vi "Func_DropMultiTypeVIs.vi"(8 "error in":errorcluster, 11 "Control Path":path=path "C:/Users/dsmith.AMER/Desktop/ctl1.ctl") -> (0 "error out":errorcluster)   [LabVIEW 2010, in "TemplateGenerator.lvlib"]
uses:
  TemplateGenerator.lvlib
  <vilib>/Utility/traverseref.llb/VI Scripting - Traverse.lvlib
  <vilib>/Utility/traverseref.llb/TRef TravTarget.ctl
  <vilib>/Utility/miscctls.llb/LVPointTypeDef.ctl
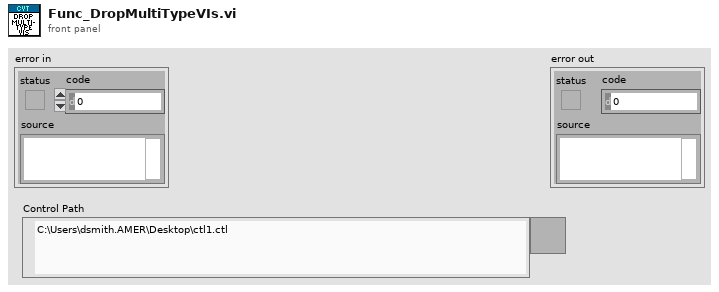
[diagram p1: front panel]
types:
  T1 = typedef "TRef TravTarget.ctl" = enum16{"FP", "BD", "Other"}
  T2 = typedef "LVPointTypeDef.ctl" = cluster{"Horizontal":i16, "Vertical":i16}
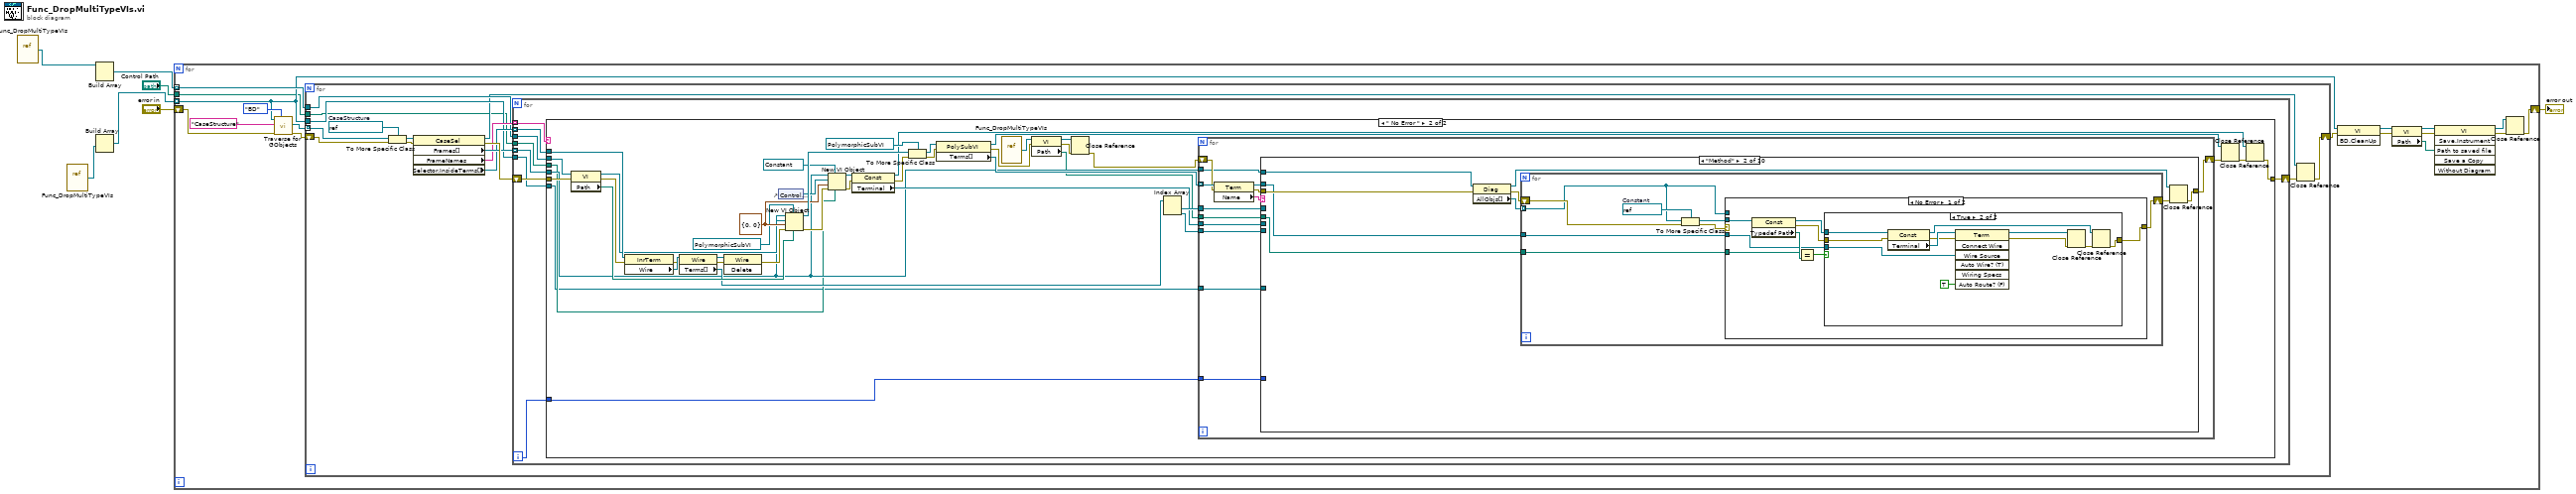
[diagram p0: block diagram]
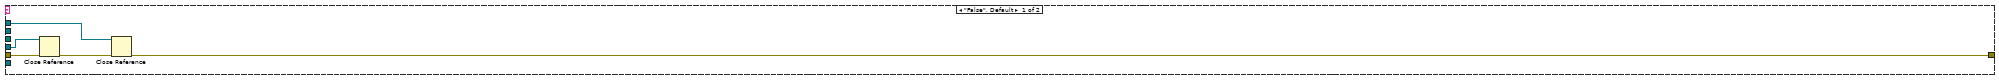
[diagram p2: hidden frame]
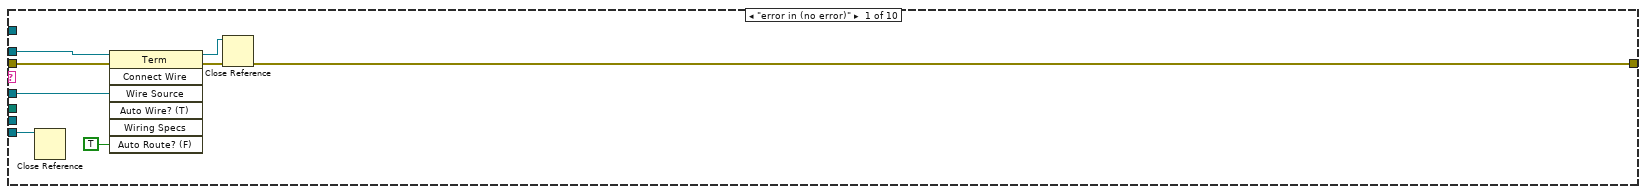
[diagram p3: hidden frame]
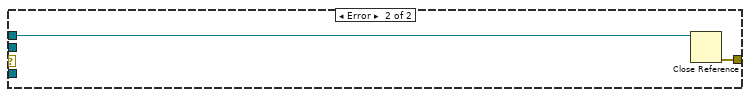
[diagram p5: hidden frame]
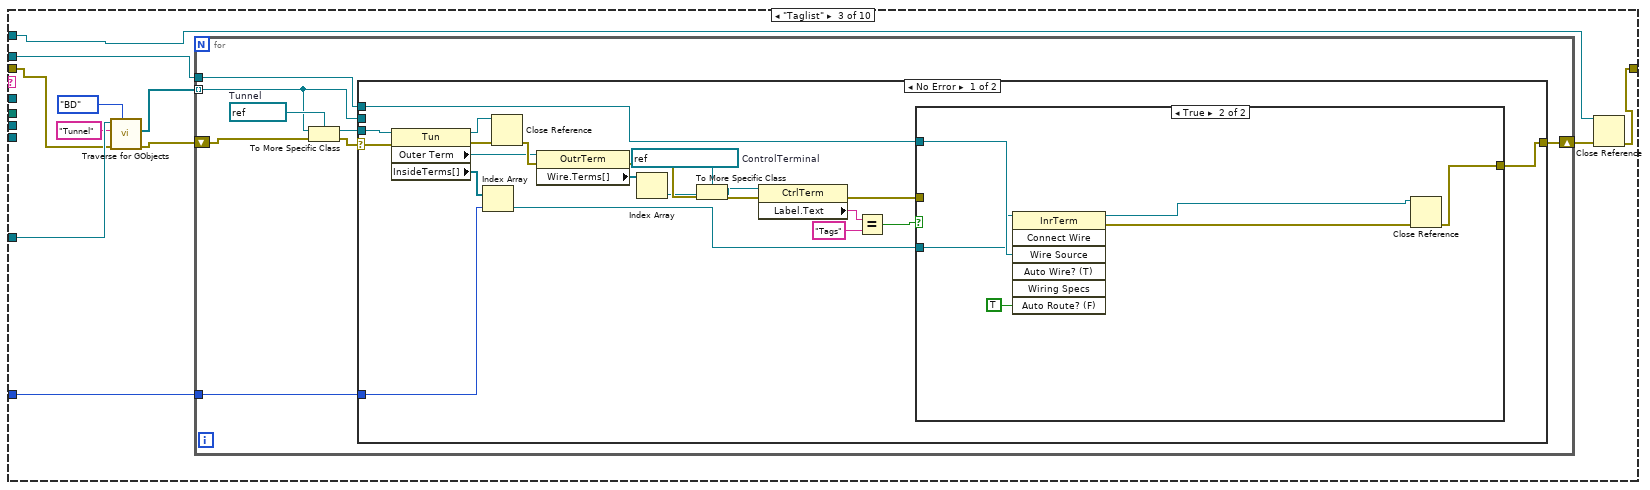
[diagram p6: hidden frame]
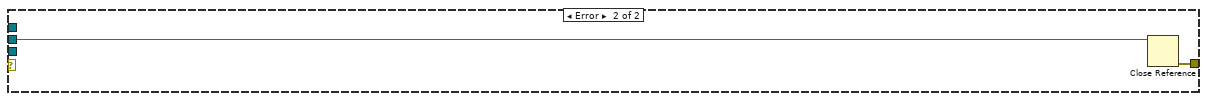
[diagram p8: hidden frame]
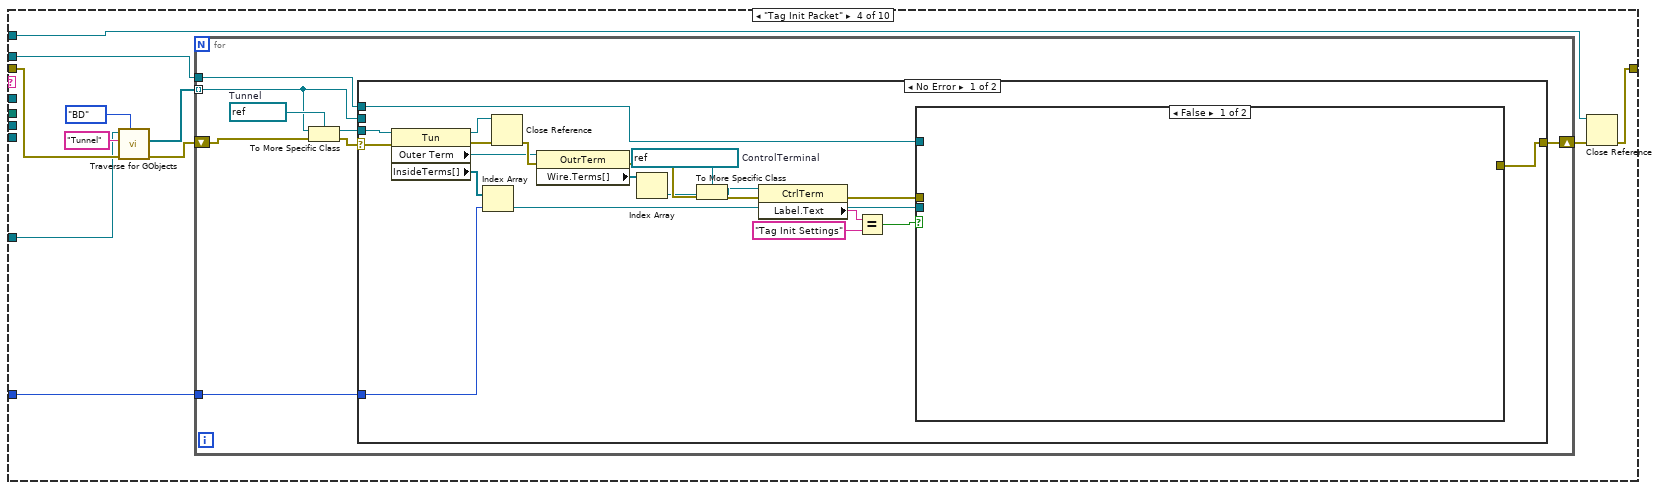
[diagram p9: hidden frame]
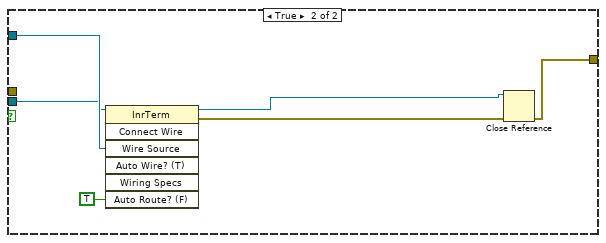
[diagram p10: hidden frame]
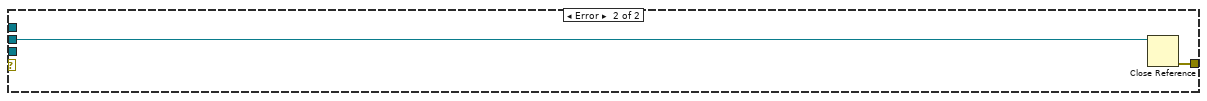
[diagram p11: hidden frame]
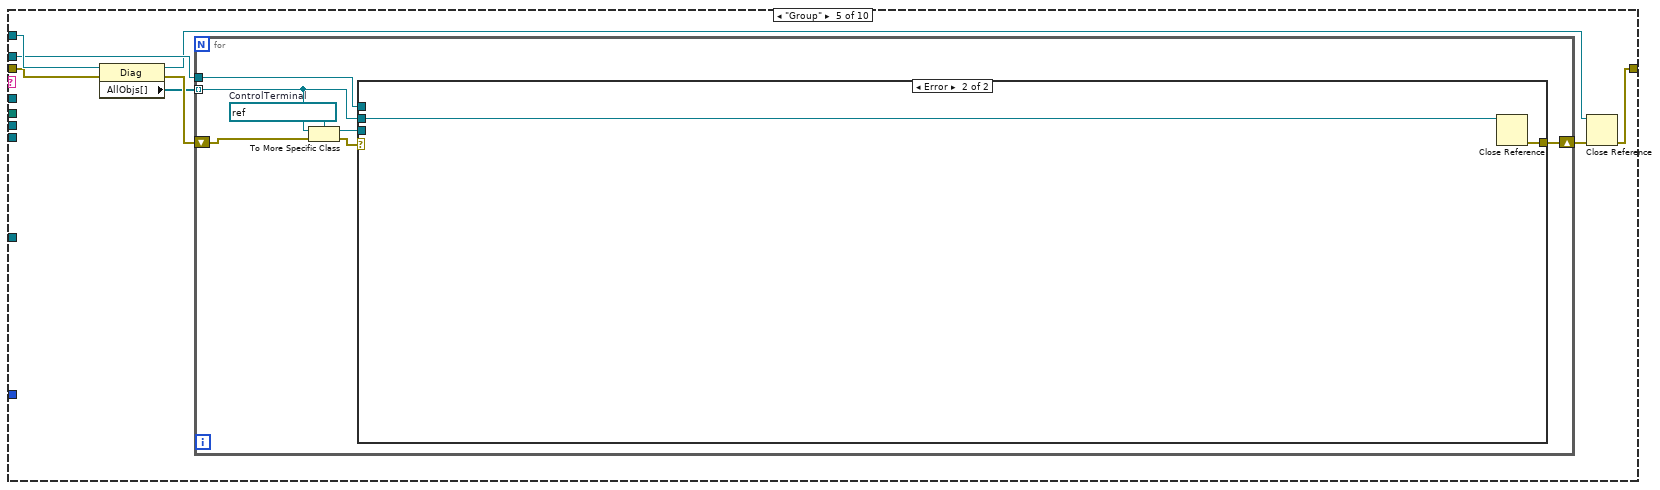
[diagram p12: hidden frame]
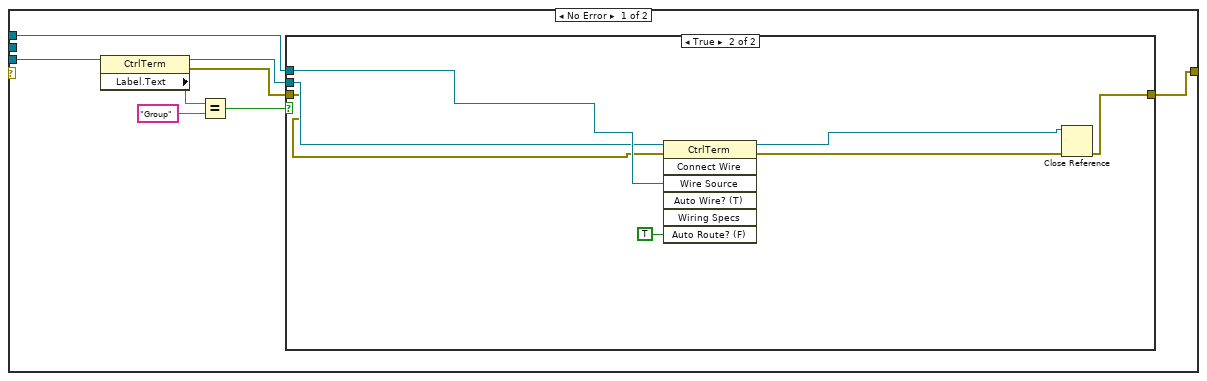
[diagram p13: hidden frame]
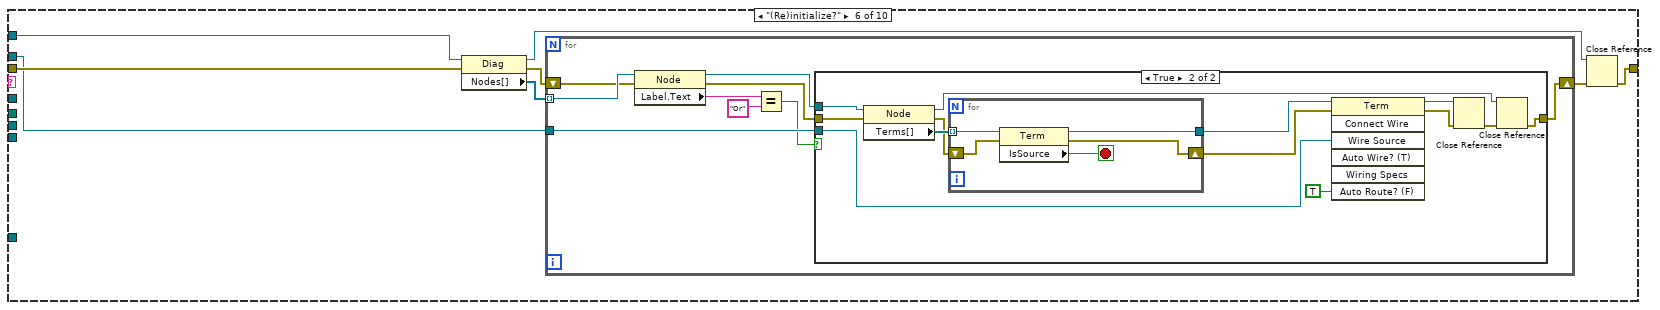
[diagram p15: hidden frame]
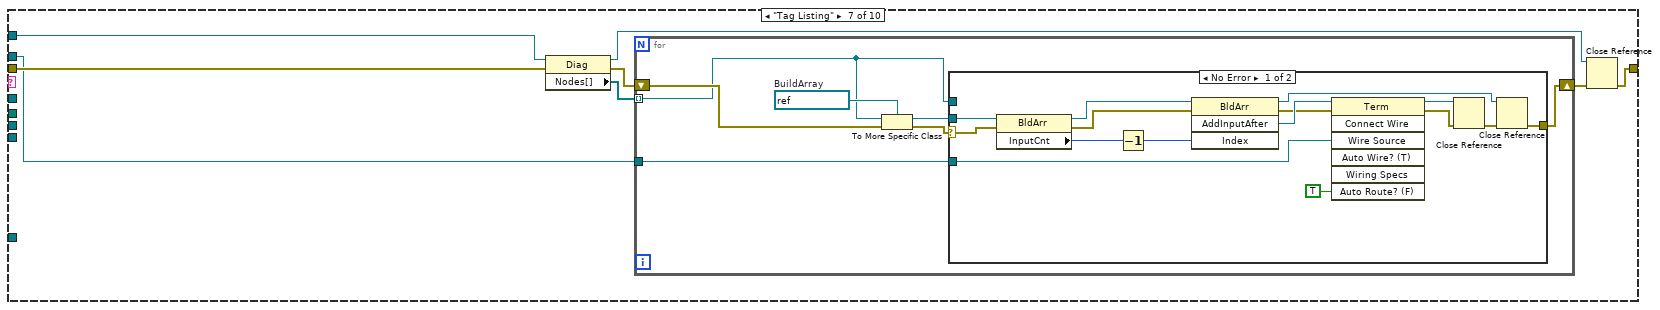
[diagram p17: hidden frame]
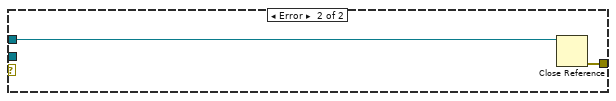
[diagram p18: hidden frame]
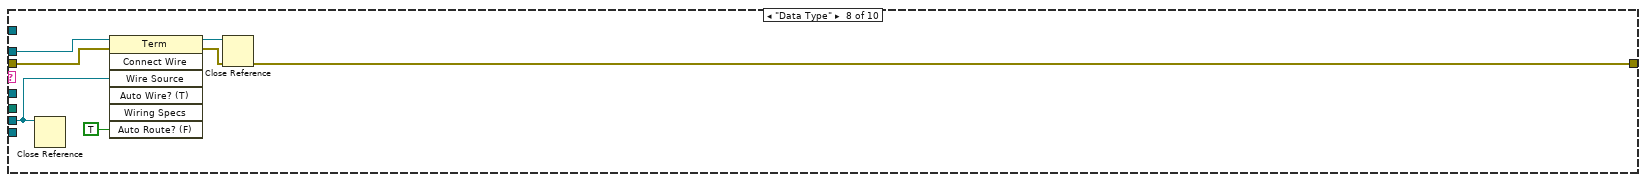
[diagram p19: hidden frame]
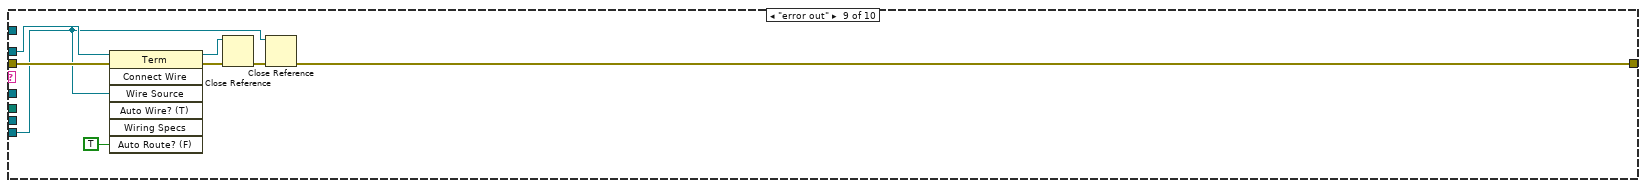
[diagram p20: hidden frame]
diagram:
  n1 = vi-ref "Func_DropMultiTypeVIs.vi"() -> (w1:refnum<vi>)
  n2 = vi-ref "Func_DropMultiTypeVIs.vi"() -> (w4:refnum<vi>)
  n3 = Build Array(w1) -> (w2:refnum<vi>[])  [unwired: 3 in]
  n4 = Build Array(w4) -> (w3:refnum<vi>[])  [unwired: 3 in]
  n5 = for {
    tunnel: w3 -> [w16] mode=indexing
    tunnel: w2 -> [w19] mode=indexing
    shift-right: [w17] -> w6
    shift-left: "error in" -> [w20]
    tunnel: "Control Path" -> [w15]
    n6 = call <vilib>:"Traverse for GObjects.vi"("Traverse Target"=TRef_TravTarget."BD", "error in (no error)"=w20, "Class Name"="CaseStructure", "VI Refnum"=w16) -> ("error out"=w23:errorcluster, "References"=w22:refnum<vi>[])  [unwired: 4 in, 2 out]
    n7 = for {
      tunnel: w22 -> [w38] mode=indexing
      tunnel: w16 -> [w30]
      shift-right: [w27] -> w18
      shift-left: w23 -> [w39]
      tunnel: w19 -> [w29]
      tunnel: w15 -> [w25]
      w37 = refnum<vi> refnum  # CaseStructure
      n8 = To More Specific Class(target class=w37, reference=w38, error in=w39) -> (specific class reference=w36:refnum<vi>, error out=w35:errorcluster)
      n9 = property class="CaseSel"(reference=w36, error in=w35) -> (reference out=w26:refnum<vi>, error out=w34:errorcluster, "Frames[]"=w33:refnum<vi>[], "FrameNames"=w32:string[], "Selector.InsideTerms[]"=w31:refnum<vi>[])
      n10 = for {
        shift-right: [w47] -> w28
        shift-left: w34 -> [w46]
        tunnel: w33 -> [w44] mode=indexing
        tunnel: w32 -> [w48] mode=indexing
        tunnel: w31 -> [w45] mode=indexing
        tunnel: w30 -> [w43]
        tunnel: w29 -> [w42]
        tunnel: w25 -> [w41]
        i -> [w40]
        n11 = case shown="\" No Error \"" w48 {
          tunnel: [w51 w58] -> w47
          tunnel: w46 -> [w53 w96]
          tunnel: w45 -> [w50 w95]
          tunnel: w44 -> [w49 w68]
          tunnel: w43 -> [_ w54]
          tunnel: w42 -> [_ w93]
          tunnel: w41 -> [_ w57]
          tunnel: w40 -> [_ w55]
          frame "False", Default {
            n12 = Close Reference(reference=w49, error in (no error)=w53) -> (error out=w52:errorcluster)
            n13 = Close Reference(reference=w50, error in (no error)=w52) -> (error out=w51:errorcluster)
          }
          frame " No Error " {
            w78 = T2 {"Horizontal"=0, "Vertical"=0} ("location")
            n14 = property class="VI"(reference=w93, error in=w96) -> (reference out=w76:refnum<vi>, error out=w94:errorcluster, "Path"=w91:path)
            n15 = property class="InrTerm"(reference=w95, error in=w94) -> (error out=w75:errorcluster, "Wire"=w90:refnum<vi>)  [unwired: 1 out]
            n16 = property class="Wire"(reference=w90, error in=w75) -> (reference out=w89:refnum<vi>, error out=w88:errorcluster, "Terms[]"=w85:refnum<vi>[])
            n17 = invoke class="Wire" method="Delete"(reference=w89, error in=w88) -> (error out=w87:errorcluster)  [unwired: 1 in, 2 out]
            n18 = control-ref of="Control Path"() -> (w72:refnum<vi>)
            n19 = New VI Object(vi object class=refnum<vi> refnum ("reference"), owner refnum=w68, style=w76, position/next to=w78, 6:w91, 8:w87) -> (object refnum=w83:refnum<vi>, 0:w86:errorcluster)  [unwired: 2 in]
            n20 = New VI Object(vi object class=refnum<vi> refnum ("reference"), owner refnum=w68, style=w72, position/next to=w78, 6:w57, 8:w86) -> (object refnum=w73:refnum<vi>, 0:w71:errorcluster)  [unwired: 2 in]
            n21 = property class="Const"(reference=w73, error in=w71) -> (reference out=w60:refnum<vi>, error out=w70:errorcluster, "Terminal"=w69:refnum<vi>)
            n22 = To More Specific Class(target class=refnum<vi> refnum ("reference"), reference=w83, error in=w70) -> (specific class reference=w82:refnum<vi>, error out=w81:errorcluster)
            n23 = property class="PolySubVI"(reference=w82, error in=w81) -> (reference out=w61:refnum<vi>, error out=w63:errorcluster, "Terms[]"=w92:refnum<vi>[])
            n24 = vi-ref "Func_DropMultiTypeVIs.vi"() -> (w67:refnum<vi>)
            n25 = property class="VI"(reference=w67, error in=w63) -> (reference out=w65:refnum<vi>, error out=w64:errorcluster, "Path"=w66:path)
            n26 = Close Reference(reference=w65, error in (no error)=w64) -> (error out=w56:errorcluster)
            n27 = Index Array(array=w85) -> (element #1=w80:refnum<vi>, element #2=w79:refnum<vi>)  [unwired: 2 in]
            n28 = for {
              shift-right: [w104] -> w62
              shift-left: w56 -> [w108]
              tunnel: w92 -> [w109] mode=indexing
              tunnel: w80 -> [w103]
              tunnel: w79 -> [w102]
              tunnel: w69 -> [w101]
              tunnel: w68 -> [w100]
              tunnel: w66 -> [w99]
              tunnel: w55 -> [w98]
              tunnel: w54 -> [w97]
              n29 = property class="Term"(reference=w109, error in=w108) -> (reference out=w105:refnum<vi>, error out=w106:errorcluster, "Name"=w107:string)
              n30 = case shown="\"Method\"" w107 {
                tunnel: [w111 w120 w158 w212 w254 w287 w323 w355 w362 w369] -> w104
                tunnel: w106 -> [w116 w125 w160 w207 w259 w292 w328 w359 w367 w369]
                tunnel: w105 -> [w117 w122 w167 w214 w256 w289 w325 w360 w368 _]
                tunnel: w103 -> [w115 _ _ _ _ _ _ _ _ _]
                tunnel: w102 -> [w110 _ _ _ _ _ _ _ w361 _]
                tunnel: w101 -> [_ _ _ _ _ _ _ w354 _ _]
                tunnel: w100 -> [_ w126 w157 w215 w260 w293 w329 _ _ _]
                tunnel: w99 -> [_ w118 _ _ _ _ _ _ _ _]
                tunnel: w98 -> [_ _ w166 w211 _ _ _ _ _ _]
                tunnel: w97 -> [_ _ w164 w205 _ _ _ _ _ _]
                frame "error in (no error)" {
                  n31 = Close Reference(reference=w110) -> ()  [unwired: 1 in, 1 out]
                  n32 = invoke class="Term" method="Connect Wire"(reference=w117, error in=w116, "Wire Source"=w115, "Auto Route? (F)"=TRUE) -> (reference out=w112:refnum<vi>, error out=w113:errorcluster)  [unwired: 3 in, 5 out]
                  n33 = Close Reference(reference=w112, error in (no error)=w113) -> (error out=w111:errorcluster)
                }
                frame "Method" {
                  n34 = property class="Diag"(reference=w126, error in=w125) -> (reference out=w119:refnum<vi>, error out=w124:errorcluster, "AllObjs[]"=w123:refnum<vi>[])
                  n35 = for {
                    shift-right: [w130] -> w121
                    shift-left: w124 -> [w132]
                    tunnel: w123 -> [w128] mode=indexing
                    tunnel: w122 -> [w129]
                    tunnel: w118 -> [w127]
                    w134 = refnum<vi> refnum  # Constant
                    n36 = To More Specific Class(target class=w134, reference=w128, error in=w132) -> (specific class reference=w133:refnum<vi>, error out=w131:errorcluster)
                    n37 = case shown="No Error" w131 {
                      tunnel: w133 -> [w142 _]
                      tunnel: [w136 w155] -> w130
                      tunnel: w129 -> [w137 _]
                      tunnel: w128 -> [_ w156]
                      tunnel: w127 -> [w135 _]
                      frame No Error {
                        n38 = property class="Const"(reference=w142) -> (reference out=w139:refnum<vi>, error out=w138:errorcluster, "Typedef Path"=w141:path)  [unwired: 1 in]
                        n39 = Equal?(x=w135, y=w141) -> (x = y?=w140:bool)
                        n40 = case shown="True" w140 {
                          tunnel: w139 -> [_ w154]
                          tunnel: w138 -> [w143 w153]
                          tunnel: w137 -> [_ w150]
                          tunnel: [w143 w144] -> w136
                          frame False {
                          }
                          frame True {
                            n41 = property class="Const"(reference=w154, error in=w153) -> (reference out=w145:refnum<vi>, error out=w151:errorcluster, "Terminal"=w152:refnum<vi>)
                            n42 = invoke class="Term" method="Connect Wire"(reference=w152, error in=w151, "Wire Source"=w150, "Auto Route? (F)"=TRUE) -> (reference out=w148:refnum<vi>, error out=w147:errorcluster)  [unwired: 3 in, 5 out]
                            n43 = Close Reference(reference=w148, error in (no error)=w147) -> (error out=w146:errorcluster)
                            n44 = Close Reference(reference=w145, error in (no error)=w146) -> (error out=w144:errorcluster)
                          }
                        }
                      }
                      frame Error {
                        n45 = Close Reference(reference=w156) -> (error out=w155:errorcluster)  [unwired: 1 in]
                      }
                    }
                  }
                  n46 = Close Reference(reference=w119, error in (no error)=w121) -> (error out=w120:errorcluster)
                }
                frame "Taglist" {
                  n47 = call <vilib>:"Traverse for GObjects.vi"("Traverse Target"=TRef_TravTarget."BD", "error in (no error)"=w160, "Class Name"="Tunnel", "VI Refnum"=w164) -> ("error out"=w161:errorcluster, "References"=w162:refnum<vi>[])  [unwired: 4 in, 2 out]
                  n48 = for {
                    shift-right: [w171] -> w159
                    shift-left: w161 -> [w173]
                    tunnel: w162 -> [w169] mode=indexing
                    tunnel: w167 -> [w170]
                    tunnel: w166 -> [w168]
                    w175 = refnum<vi> refnum  # Tunnel
                    n49 = To More Specific Class(target class=w175, reference=w169, error in=w173) -> (specific class reference=w174:refnum<vi>, error out=w172:errorcluster)
                    n50 = case shown="No Error" w172 {
                      selector: w172 -> [w193 _]
                      tunnel: w174 -> [w196 _]
                      tunnel: [w194 w203] -> w171
                      tunnel: w170 -> [w195 _]
                      tunnel: w169 -> [_ w204]
                      tunnel: w168 -> [w191 _]
                      frame No Error {
                        w182 = refnum<vi> refnum  # ControlTerminal
                        n51 = property class="Tun"(reference=w196, error in=w193) -> (reference out=w189:refnum<vi>, error out=w188:errorcluster, "Outer Term"=w186:refnum<vi>, "InsideTerms[]"=w192:refnum<vi>[])
                        n52 = Index Array(array=w192, index=w191) -> (element=w190:refnum<vi>)
                        n53 = Close Reference(reference=w189, error in (no error)=w188) -> (error out=w187:errorcluster)
                        n54 = property class="OutrTerm"(reference=w186, error in=w187) -> (error out=w184:errorcluster, "Wire.Terms[]"=w185:refnum<vi>[])  [unwired: 1 out]
                        n55 = Index Array(array=w185) -> (element=w183:refnum<vi>)  [unwired: 1 in]
                        n56 = To More Specific Class(target class=w182, reference=w183, error in=w184) -> (specific class reference=w181:refnum<vi>, error out=w180:errorcluster)
                        n57 = property class="CtrlTerm"(reference=w181, error in=w180) -> (error out=w176:errorcluster, "Label.Text"=w179:string)  [unwired: 1 out]
                        n58 = Equal?(x=w179, y="Tags") -> (x = y?=w177:bool)
                        n59 = case shown="True" w177 {
                          tunnel: w195 -> [_ w202]
                          tunnel: [_ w199] -> w194
                          tunnel: w190 -> [_ w197]
                          tunnel: w176 -> [_ _]
                          frame False {
                          }
                          frame True {
                            n60 = invoke class="InrTerm" method="Connect Wire"(reference=w197, "Wire Source"=w202, "Auto Route? (F)"=TRUE) -> (reference out=w201:refnum<vi>, error out=w200:errorcluster)  [unwired: 4 in, 5 out]
                            n61 = Close Reference(reference=w201, error in (no error)=w200) -> (error out=w199:errorcluster)
                          }
                        }
                      }
                      frame Error {
                        n62 = Close Reference(reference=w204) -> (error out=w203:errorcluster)  [unwired: 1 in]
                      }
                    }
                  }
                  n63 = Close Reference(reference=w157, error in (no error)=w159) -> (error out=w158:errorcluster)
                }
                frame "Tag Init Packet" {
                  n64 = call <vilib>:"Traverse for GObjects.vi"("Traverse Target"=TRef_TravTarget."BD", "error in (no error)"=w207, "Class Name"="Tunnel", "VI Refnum"=w205) -> ("error out"=w208:errorcluster, "References"=w206:refnum<vi>[])  [unwired: 4 in, 2 out]
                  n65 = for {
                    shift-right: [w219] -> w213
                    shift-left: w208 -> [w221]
                    tunnel: w206 -> [w217] mode=indexing
                    tunnel: w214 -> [w218]
                    tunnel: w211 -> [w216]
                    w223 = refnum<vi> refnum  # Tunnel
                    n66 = To More Specific Class(target class=w223, reference=w217, error in=w221) -> (specific class reference=w222:refnum<vi>, error out=w220:errorcluster)
                    n67 = case shown="No Error" w220 {
                      selector: w220 -> [w241 _]
                      tunnel: w222 -> [w244 _]
                      tunnel: [w242 w251] -> w219
                      tunnel: w218 -> [w243 _]
                      tunnel: w217 -> [_ w252]
                      tunnel: w216 -> [w239 _]
                      frame No Error {
                        w230 = refnum<vi> refnum  # ControlTerminal
                        n68 = property class="Tun"(reference=w244, error in=w241) -> (reference out=w237:refnum<vi>, error out=w236:errorcluster, "Outer Term"=w234:refnum<vi>, "InsideTerms[]"=w240:refnum<vi>[])
                        n69 = Index Array(array=w240, index=w239) -> (element=w238:refnum<vi>)
                        n70 = Close Reference(reference=w237, error in (no error)=w236) -> (error out=w235:errorcluster)
                        n71 = property class="OutrTerm"(reference=w234, error in=w235) -> (error out=w232:errorcluster, "Wire.Terms[]"=w233:refnum<vi>[])  [unwired: 1 out]
                        n72 = Index Array(array=w233) -> (element=w231:refnum<vi>)  [unwired: 1 in]
                        n73 = To More Specific Class(target class=w230, reference=w231, error in=w232) -> (specific class reference=w229:refnum<vi>, error out=w228:errorcluster)
                        n74 = property class="CtrlTerm"(reference=w229, error in=w228) -> (error out=w224:errorcluster, "Label.Text"=w227:string)  [unwired: 1 out]
                        n75 = Equal?(x=w227, y="Tag Init Settings") -> (x = y?=w225:bool)
                        n76 = case shown="False" w225 {
                          tunnel: w243 -> [_ w250]
                          tunnel: [_ w247] -> w242
                          tunnel: w238 -> [_ w245]
                          tunnel: w224 -> [_ _]
                          frame False {
                          }
                          frame True {
                            n77 = invoke class="InrTerm" method="Connect Wire"(reference=w245, "Wire Source"=w250, "Auto Route? (F)"=TRUE) -> (reference out=w249:refnum<vi>, error out=w248:errorcluster)  [unwired: 4 in, 5 out]
                            n78 = Close Reference(reference=w249, error in (no error)=w248) -> (error out=w247:errorcluster)
                          }
                        }
                      }
                      frame Error {
                        n79 = Close Reference(reference=w252) -> (error out=w251:errorcluster)  [unwired: 1 in]
                      }
                    }
                  }
                  n80 = Close Reference(reference=w215, error in (no error)=w213) -> (error out=w212:errorcluster)
                }
                frame "Group" {
                  n81 = property class="Diag"(reference=w260, error in=w259) -> (reference out=w253:refnum<vi>, error out=w258:errorcluster, "AllObjs[]"=w257:refnum<vi>[])
                  n82 = for {
                    shift-right: [w263] -> w255
                    shift-left: w258 -> [w265]
                    tunnel: w257 -> [w261] mode=indexing
                    tunnel: w256 -> [w262]
                    w267 = refnum<vi> refnum  # ControlTerminal
                    n83 = To More Specific Class(target class=w267, reference=w261, error in=w265) -> (specific class reference=w266:refnum<vi>, error out=w264:errorcluster)
                    n84 = case shown="Error" w264 {
                      tunnel: w266 -> [w275 _]
                      tunnel: [w270 w284] -> w263
                      tunnel: w262 -> [w271 _]
                      tunnel: w261 -> [_ w285]
                      frame No Error {
                        n85 = property class="CtrlTerm"(reference=w275) -> (reference out=w273:refnum<vi>, error out=w272:errorcluster, "Label.Text"=w269:string)  [unwired: 1 in]
                        n86 = Equal?(x=w269, y="Group") -> (x = y?=w274:bool)
                        n87 = case shown="True" w274 {
                          tunnel: w273 -> [_ w279]
                          tunnel: w272 -> [w276 w278]
                          tunnel: w271 -> [_ w283]
                          tunnel: [w276 w280] -> w270
                          frame False {
                          }
                          frame True {
                            n88 = invoke class="CtrlTerm" method="Connect Wire"(reference=w279, error in=w278, "Wire Source"=w283, "Auto Route? (F)"=TRUE) -> (reference out=w282:refnum<vi>, error out=w281:errorcluster)  [unwired: 3 in, 5 out]
                            n89 = Close Reference(reference=w282, error in (no error)=w281) -> (error out=w280:errorcluster)
                          }
                        }
                      }
                      frame Error {
                        n90 = Close Reference(reference=w285) -> (error out=w284:errorcluster)  [unwired: 1 in]
                      }
                    }
                  }
                  n91 = Close Reference(reference=w253, error in (no error)=w255) -> (error out=w254:errorcluster)
                }
                frame "(Re)initialize?" {
                  n92 = property class="Diag"(reference=w293, error in=w292) -> (reference out=w286:refnum<vi>, error out=w291:errorcluster, "Nodes[]"=w290:refnum<vi>[])
                  n93 = for {
                    shift-right: [w302] -> w288
                    shift-left: w291 -> [w294]
                    tunnel: w290 -> [w300] mode=indexing
                    tunnel: w289 -> [w301]
                    n94 = property class="Node"(reference=w300, error in=w294) -> (reference out=w298:refnum<vi>, error out=w297:errorcluster, "Label.Text"=w296:string)
                    n95 = Equal?(x=w296, y="Or") -> (x = y?=w299:bool)
                    n96 = case shown="True" w299 {
                      tunnel: w298 -> [_ w316]
                      tunnel: w297 -> [w303 w315]
                      tunnel: w301 -> [_ w314]
                      tunnel: [w303 w308] -> w302
                      frame False {
                      }
                      frame True {
                        n97 = property class="Node"(reference=w316, error in=w315) -> (reference out=w309:refnum<vi>, error out=w306:errorcluster, "Terms[]"=w307:refnum<vi>[])
                        n98 = for {
                          tunnel: w307 -> [w321] mode=indexing
                          shift-right: [w319] -> w304
                          shift-left: w306 -> [w320]
                          tunnel: [w317] -> w305
                          stop <- w318 stop-if-true
                          n99 = property on="Property Node" class="Term"(reference=w321, error in=w320) -> (reference out=w317:refnum<vi>, error out=w319:errorcluster, "IsSource"=w318:bool)
                        }
                        n100 = invoke class="Term" method="Connect Wire"(reference=w305, error in=w304, "Wire Source"=w314, "Auto Route? (F)"=TRUE) -> (reference out=w312:refnum<vi>, error out=w311:errorcluster)  [unwired: 3 in, 5 out]
                        n101 = Close Reference(reference=w312, error in (no error)=w311) -> (error out=w310:errorcluster)
                        n102 = Close Reference(reference=w309, error in (no error)=w310) -> (error out=w308:errorcluster)
                      }
                    }
                  }
                  n103 = Close Reference(reference=w286, error in (no error)=w288) -> (error out=w287:errorcluster)
                }
                frame "Tag Listing" {
                  n104 = property class="Diag"(reference=w329, error in=w328) -> (reference out=w322:refnum<vi>, error out=w327:errorcluster, "Nodes[]"=w326:refnum<vi>[])
                  n105 = for {
                    shift-right: [w332] -> w324
                    shift-left: w327 -> [w334]
                    tunnel: w326 -> [w330] mode=indexing
                    tunnel: w325 -> [w331]
                    w336 = refnum<vi> refnum  # BuildArray
                    n106 = To More Specific Class(target class=w336, reference=w330, error in=w334) -> (specific class reference=w335:refnum<vi>, error out=w333:errorcluster)
                    n107 = case shown="No Error" w333 {
                      selector: w333 -> [w343 _]
                      tunnel: w335 -> [w351 _]
                      tunnel: [w349 w352] -> w332
                      tunnel: w331 -> [w350 _]
                      tunnel: w330 -> [_ w353]
                      frame No Error {
                        n108 = property class="BldArr"(reference=w351, error in=w343) -> (reference out=w342:refnum<vi>, error out=w341:errorcluster, "InputCnt"=w348:i32)
                        n109 = Decrement(x=w348) -> (x-1=w340:i32)
                        n110 = invoke class="BldArr" method="AddInputAfter"(reference=w342, error in=w341, "Index"=w340) -> (reference out=w337:refnum<vi>, error out=w338:errorcluster, "AddInputAfter"=w339:refnum<vi>)  [unwired: 1 in, 1 out]
                        n111 = invoke class="Term" method="Connect Wire"(reference=w339, error in=w338, "Wire Source"=w350, "Auto Route? (F)"=TRUE) -> (reference out=w346:refnum<vi>, error out=w345:errorcluster)  [unwired: 3 in, 5 out]
                        n112 = Close Reference(reference=w346, error in (no error)=w345) -> (error out=w344:errorcluster)
                        n113 = Close Reference(reference=w337, error in (no error)=w344) -> (error out=w349:errorcluster)
                      }
                      frame Error {
                        n114 = Close Reference(reference=w353) -> (error out=w352:errorcluster)  [unwired: 1 in]
                      }
                    }
                  }
                  n115 = Close Reference(reference=w322, error in (no error)=w324) -> (error out=w323:errorcluster)
                }
                frame "Data Type" {
                  n116 = Close Reference(reference=w354) -> ()  [unwired: 1 in, 1 out]
                  n117 = invoke class="Term" method="Connect Wire"(reference=w360, error in=w359, "Wire Source"=w354, "Auto Route? (F)"=TRUE) -> (reference out=w356:refnum<vi>, error out=w357:errorcluster)  [unwired: 3 in, 5 out]
                  n118 = Close Reference(reference=w356, error in (no error)=w357) -> (error out=w355:errorcluster)
                }
                frame "error out" {
                  n119 = invoke class="Term" method="Connect Wire"(reference=w368, error in=w367, "Wire Source"=w361, "Auto Route? (F)"=TRUE) -> (reference out=w364:refnum<vi>, error out=w365:errorcluster)  [unwired: 3 in, 5 out]
                  n120 = Close Reference(reference=w364, error in (no error)=w365) -> (error out=w363:errorcluster)
                  n121 = Close Reference(reference=w361, error in (no error)=w363) -> (error out=w362:errorcluster)
                }
                frame Default {
                }
              }
            }
            n122 = Close Reference(reference=w61, error in (no error)=w62) -> (error out=w59:errorcluster)
            n123 = Close Reference(reference=w60, error in (no error)=w59) -> (error out=w58:errorcluster)
          }
        }
      }
      n124 = Close Reference(reference=w26, error in (no error)=w28) -> (error out=w27:errorcluster)
    }
    n125 = invoke class="VI" method="BD.CleanUp"(reference=w16, error in=w18) -> (reference out=w14:refnum<vi>, error out=w13:errorcluster)  [unwired: 1 in, 1 out]
    n126 = property class="VI"(reference=w14, error in=w13) -> (reference out=w12:refnum<vi>, error out=w11:errorcluster, "Path"=w10:path)
    n127 = invoke class="VI" method="Save.Instrument"(reference=w12, error in=w11, "Path to saved file"=w10) -> (reference out=w8:refnum<vi>, error out=w9:errorcluster)  [unwired: 3 in, 4 out]
    n128 = Close Reference(reference=w8, error in (no error)=w9) -> (error out=w17:errorcluster)
  }
  "error out" <- w6
